vi "Set Speed.vi"(8 "error in":errorcluster, 10 "Pump %":dbl, 11 "Tacmina Settings in":T1) -> (0 "error out":errorcluster, 1 "Connection Error":bool, 3 "Tacmina Settings out":T1)   [LabVIEW 2018, in "Tacmina QI.lvlib"]
uses:
  Tacmina QI.lvlib
  Tacmina QI DAQ Setting.ctl
  <vilib>/DAQmx/write.llb/DAQmx Write (Analog DBL 1Chan 1Samp).vi
  <vilib>/DAQmx/write.llb/DAQmx Write (Digital Bool 1Line 1Point).vi
  <vilib>/DAQmx/miscellaneous.llb/DAQmx Fill In Error Info.vi
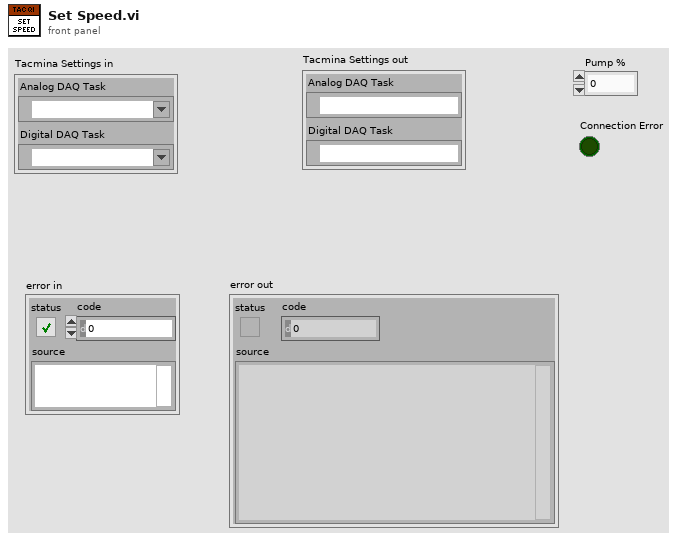
[diagram p1: front panel]
types:
  T1 = typedef "Tacmina QI.lvlib/Tacmina QI DAQ Setting.ctl" = cluster{"Analog DAQ Task":refnum<k21>, "Digital DAQ Task":refnum<k21>}
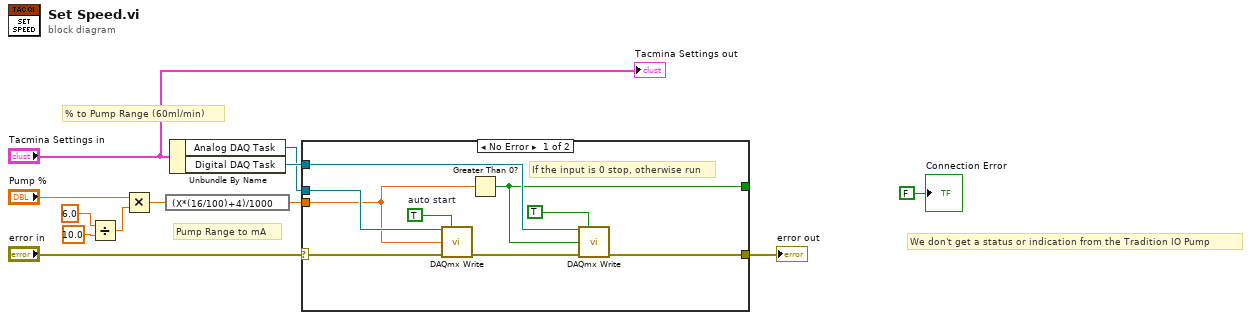
[diagram p0: block diagram]
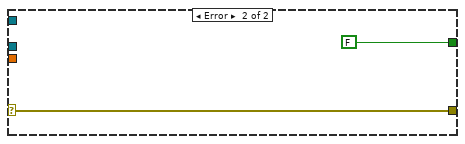
[diagram p2: hidden frame]
diagram:
  # "We don't get a status or indication from the Tradition IO Pump"
  # "% to Pump Range (60ml/min)"
  # "Pump Range to mA"
  n1 = Divide(x=6.0, y=10.0) -> (x/y=w2:dbl)
  n2 = Multiply(x="Pump %", y=w2) -> (x*y=w1:dbl)
  n3 = expression code="(X*(16/100)+4)/1000"(w1) -> (w12:dbl)
  n4 = Unbundle By Name("Tacmina Settings in") -> ("Analog DAQ Task"=w9:refnum<k21>, "Digital DAQ Task"=w10:refnum<k21>)
  n5 = case shown="No Error" "error in" {
    selector: "error in" -> [w13 w22]
    tunnel: w10 -> [w21 _]
    tunnel: w12 -> [w14 _]
    tunnel: w9 -> [w20 _]
    tunnel: [w15 w22] -> w7
    tunnel: [w17 FALSE ("Pump On?")] -> _
    frame No Error {
      w18 = TRUE  # auto start
      # "If the input is 0 stop, otherwise run"
      n6 = call-poly <vilib>:"DAQmx Write.vi"("task/channels in"=w20, "auto start"=w18, "data"=w14, "error in"=w13) -> ("error out"=w16:errorcluster)  [unwired: 9 in, 2 out]
      n7 = Greater Than 0?(x=w14) -> (x > 0?=w17:bool)
      n8 = call-poly <vilib>:"DAQmx Write.vi"("task/channels in"=w21, "auto start"=TRUE, "data"=w17, "error in"=w16) -> ("error out"=w15:errorcluster)  [unwired: 9 in, 2 out]
    }
    frame Error {
    }
  }
  "error out" <- w7
  "Tacmina Settings out" <- "Tacmina Settings in"
  "Connection Error" <- FALSE ("Connection Error")
